vi "Push String.vi"(8 "Input Boolean":bool, 11 "Input String":string) -> (3 "Output String":string)   [LabVIEW 2019]
doc: "If the Boolean in is TRUE then the \"Output String\" is the \"Input String\".\n\nIf the Boolean in is FALSE then the \"Output String\" is blank."
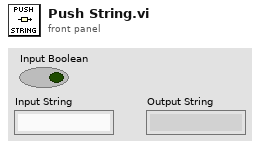
[diagram p1: front panel]
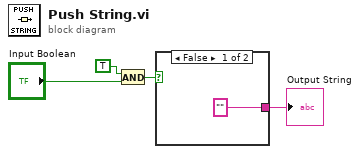
[diagram p0: block diagram]
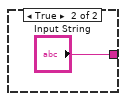
[diagram p2: hidden frame]
diagram:
  n1 = And(x=TRUE, y="Input Boolean") -> (x .and. y?=w4:bool)
  n2 = case shown="False" w4 {
    tunnel: ["" "Input String"] -> w1
    frame False {
    }
    frame True {
    }
  }
  "Output String" <- w1
